vi "Slider Control 2 Index.vi"(9 "Control":refnum<vi>, 11 "Controls":refnum<vi>[](array[refnum])) -> (2 "Index":i32)   [LabVIEW 2013]
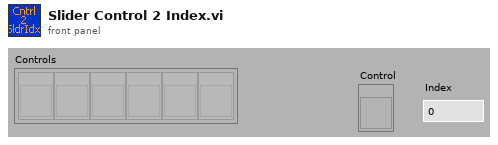
[diagram p1: front panel]
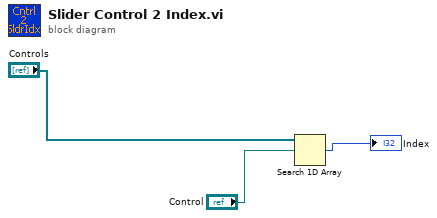
[diagram p0: block diagram]
diagram:
  n1 = Search 1D Array(1D array="Controls", element="Control") -> (index of element=→"Index":i32)  [unwired: 1 in]
